vi "I2C L76K DFRobot Gravity GPS.vi"() -> ()   [LabVIEW 2020, in "CTI-Scratchpad.lvlib"]
uses:
  CTI-Scratchpad.lvlib
  CTI/Identity.ctl
  CTI-Peripheral/GPS/DFRobot_Gravity_GNSS/Private/GPSReturn.ctl
  CTI/Error Reporting.ctl
  CTI/GPIO Number.ctl
  CTI/I2C Number.ctl
  CTI/Session/Session.lvclass
  CTI-Peripheral/GPS/DFRobot_Gravity_GNSS/DFRobot_Gravity_GNSS.lvclass
  CTI/VisaComms/VisaComms.lvclass
  CTI/CTI.lvlib
panel:
  out "string":string
  out "Open Streetmap Url":string
  out "GPSReturn":T1 {"UTC Time Stamp" format="%<%.3X>T"; "Longitude" format="%#_12f"; "Latitude" format="%#_12f"}
  in  "Stop":bool
  out "loop":i32
  out "Identity":T2
  in  "Grove Connector":enum16{"I2C0", "I2C1"}(ring)
  out "error out":errorcluster
  in  "Port":refnum<visa-resource-name>="COM4"
  # "https://wiki.dfrobot.com/tel0157"
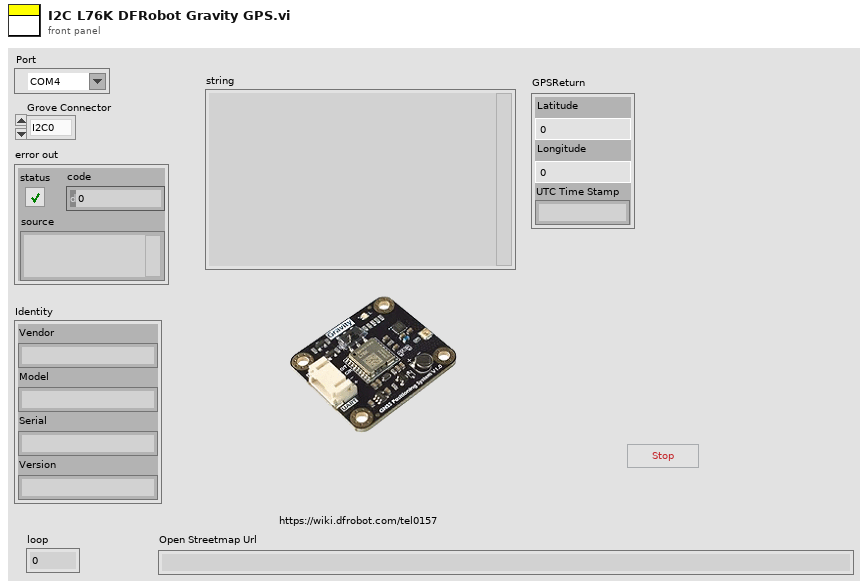
[diagram p1: front panel]
types:
  T1 = typedef "CTI-Peripheral.lvlib/DFRobot_Gravity_GNSS.lvclass/GPSReturn.ctl" = cluster{"Latitude":dbl, "Longitude":dbl, "UTC Time Stamp":timestamp}
  T2 = typedef "CTI.lvlib/Identity.ctl" = cluster{"Vendor":string, "Model":string, "Serial":string, "Version":string}
  T3 = typedef "CTI.lvlib/Error Reporting.ctl" = enum16{"Minimal", "Moderate", "Full"}
  T4 = typedef "CTI.lvlib/I2C Number.ctl" = i8
  T5 = typedef "CTI.lvlib/GPIO Number.ctl" = i8
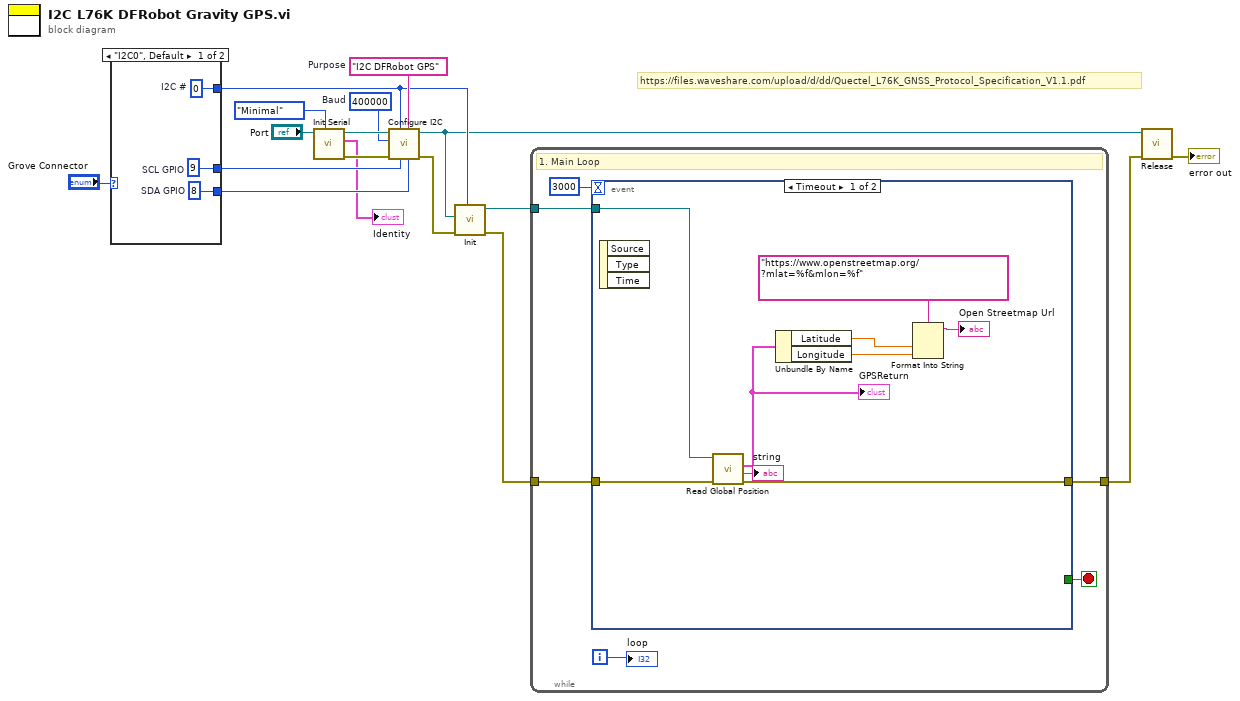
[diagram p0: block diagram]
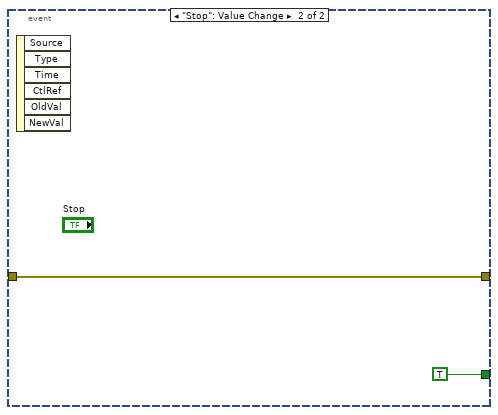
[diagram p2: hidden frame]
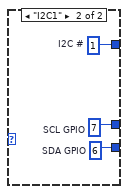
[diagram p3: hidden frame]
diagram:
  w12 = "I2C DFRobot GPS"  # Purpose
  w13 = u32 400000  # Baud
  # "https://files.waveshare.com/upload/d/dd/Quectel_L76K_GNSS_Protocol_Specification_V1.1.pdf"
  n1 = case shown="\"I2C0\", Default" "Grove Connector" {
    tunnel: [w20 w23] -> w10
    tunnel: [w19 w22] -> w9
    tunnel: [w18 w21] -> w5
    frame "I2C0", Default {
      w18 = T4 0  # I2C #
      w19 = T5 8  # SDA GPIO
      w20 = T5 9  # SCL GPIO
    }
    frame "I2C1" {
      w21 = T4 1  # I2C #
      w22 = T5 6  # SDA GPIO
      w23 = T5 7  # SCL GPIO
    }
  }
  n2 = call "Init Serial.vi"("Error Checking (Full)"=Error_Reporting."Minimal", "VISA resource name in"="Port") -> ("error out"=w14:errorcluster, "Identity"=→"Identity":T2, "Session"=w15:refnum<class "Session.lvclass">)  [unwired: 7 in]
  n3 = call "Configure I2C.vi"("SDA GPIO"=w9, "Purpose (\"I2C\")"=w12, "SCL GPIO"=w10, "I2C #"=w5, "error in (no error)"=w14, "Baud"=w13, "Session in"=w15) -> ("error out"=w3:errorcluster, "Session out"=w4:refnum<class "Session.lvclass">)  [unwired: 3 in]
  n4 = call "Init.vi"("I2C #"=w5, "error in (no error)"=w3, "Session In"=w4) -> ("error out"=w2:errorcluster, "DFRobot_Gravity_GNSS Out"=w1:refnum<class "DFRobot_Gravity_GNSS.lvclass">)  [unwired: 7 in]
  n5 = while {
    tunnel: w2 -> [w28]
    tunnel: w1 -> [w29]
    tunnel: [w26] -> w7
    i -> [w27]
    stop <- w24 stop-if-true
    # "1. Main Loop"
    n6 = event shown="[0] Timeout" {
      selector: _ -> [_ _]
      dyn-events: _ -> [_ _]
      timeout: 3000 -> [_ _]
      tunnel: w29 -> [w36 _]
      tunnel: w28 -> [w37 w39]
      tunnel: [w38 w39] -> w26
      tunnel: [_ TRUE] -> w24
      event Timeout {
        n7 = event-data() -> ()  [unwired: 1 in, 3 out]
        n8 = call-dynamic "Read Global Position.vi"("error in (no error)"=w37, "DFRobot_Gravity_GNSS in"=w36) -> ("error out"=w38:errorcluster, "string"=→"string":string, "GPSReturn"=w33:T1)  [unwired: 6 in, 1 out]
        "GPSReturn" <- w33
        n9 = Unbundle By Name(w33) -> ("Latitude"=w32:dbl, "Longitude"=w31:dbl)
        n10 = Format Into String(format string="https://www.openstreetmap.org/?mlat=%f&mlon=%f", w32, w31) -> (resulting string=→"Open Streetmap Url":string)  [unwired: 2 in, 1 out]
      }
      event "Stop": Value Change {
        n11 = event-data() -> ()  [unwired: 1 in, 6 out]
      }
    }
    "loop" <- w27
  }
  n12 = call-dynamic "Release.vi"("error in (no error)"=w7, "Session in"=w4) -> ("error out"=→"error out":errorcluster)  [unwired: 9 in]
